vi "design V6.vi"() -> ()   [LabVIEW 2018]
panel:
  in  "set angle! 2":dbl(slide)=-33.45836363636363 scale=346.0..51.0
  in  "set step ! 4":dbl(slide)=6549.0 min=0.0 max=16000.0 step=1.0 scale=94.0..64.0
  in  "current dial":dbl format="%_2f"
  in  "setup":bool
  in  "calibration (deg/step)":dbl format="%_2f"
  in  "probe id":enum16{""}(ring)
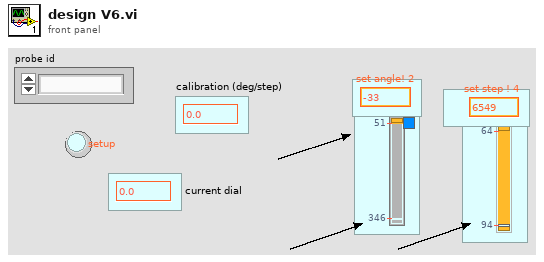
[diagram p1: front panel]
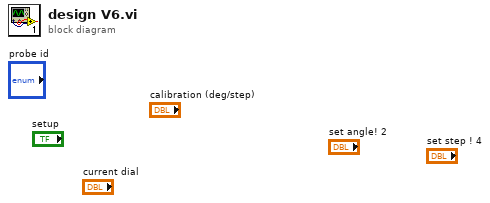
[diagram p0: block diagram]
diagram:
